vi "OFDMTX.vi"(2 "Transmitter Properties":T1 {"Window" items=["Rectangular", "Bohman", "Parzen", "Bartlett-Hanning", "Blackman-Nuttall", "Blackman", "Hanning", "Hamming", "Welch", "Exact Blackman", "Blackman-Harris", "Triangle"]}, 3 "Generate Training Symbol":bool, 4 "Input Bits":bool[](array[boolean])) -> (1 "output cluster":cluster{dbl, dbl, "Time Domain Out":cdb[]})   [LabVIEW 2020]
doc: "Takes in a group of bits as well as various parameters, and outputs a complex baseband OFDM symbol. Note that if an odd number of subcarriers is used, the carrier power parameter is ignored. For more help on the individual parameters and modules, check the relevant sub-VIs."
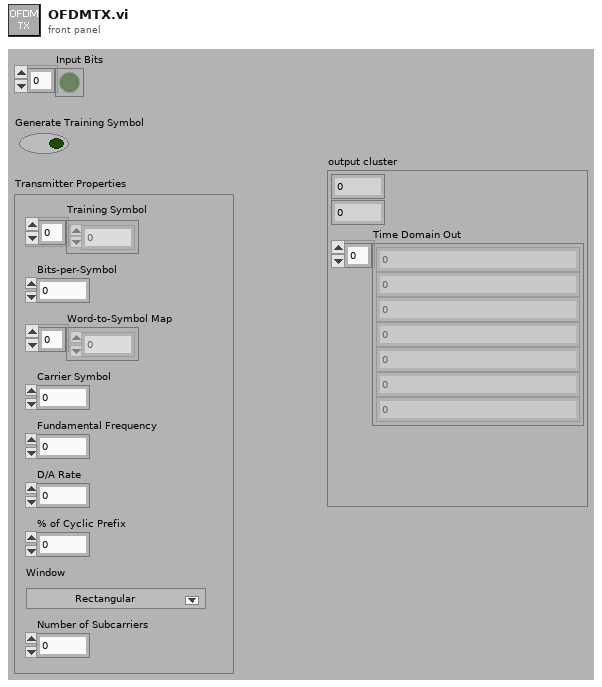
[diagram p1: front panel]
types:
  T1 = cluster{"Word-to-Symbol Map":cdb[], "% of Cyclic Prefix":dbl, "Training Symbol":cdb[], "Bits-per-Symbol":i32, "Carrier Symbol":cdb, "Fundamental Frequency":dbl, "D/A Rate":dbl, "Window":u16, "Number of Subcarriers":i32}
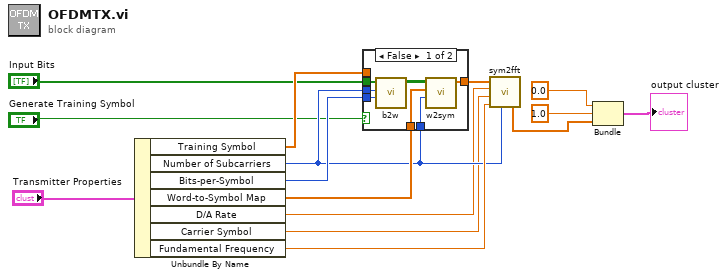
[diagram p0: block diagram]
diagram:
  n1 = Unbundle By Name("Transmitter Properties") -> ("Training Symbol"=w13:cdb[], "Number of Subcarriers"=w9:i32, "Bits-per-Symbol"=w10:i32, "Word-to-Symbol Map"=w12:cdb[], "D/A Rate"=w6:dbl, "Carrier Symbol"=w5:cdb, "Fundamental Frequency"=w11:dbl)
  n2 = case shown="False" "Generate Training Symbol" {
    tunnel: w13 -> [_ w23]
    tunnel: [w22 w23] -> w15
    tunnel: w12 -> [w20 _]
    tunnel: w9 -> [w18 _]
    tunnel: "Input Bits" -> [w19 _]
    tunnel: w10 -> [w17 _]
    tunnel: w9 -> [w16 _]
    frame False {
      n3 = call "b2w.vi"("Parallel Input"=w19, "Number of Subcarriers"=w18, "Bits-per-Symbol"=w17) -> ("Parallel Word Out"=w21:bool[][])  [unwired: 7 out]
      n4 = call "w2sym.vi"("Number of Subcarriers"=w16, "Word-to-Symbol Map"=w20, "Parallel Word Input"=w21) -> ("Parallel Symbol Output"=w22:cdb[])  [unwired: 8 out]
    }
    frame True {
    }
  }
  n5 = call "sym2fft.vi"("Number of Subcarriers"=w9, "Fundamental Frequency"=w11, "Carrier Symbol"=w5, "D/A Rate"=w6, "Parallel Symbol In"=w15) -> ("Time Domain Out"=w1:cdb[])  [unwired: 6 out]
  n6 = Bundle(0.0, 1.0, "Time Domain Out"=w1) -> (→"output cluster":cluster{dbl, dbl, "Time Domain Out":cdb[]})  [unwired: 1 in]
